vi "Send Command.vi"(8 "error in (no error)":errorcluster, 9 "timeout in ms (0)":i32 format="%d ms", 10 "command":T1={"Command"=enum."Rx", "Parameters"={"arg1"=0, "arg2"=0}}, 11 "Plugin Interface in":refnum<class "Plugin Interface.lvclass">) -> (0 "error out":errorcluster, 3 "Plugin Interface out":refnum<class "Plugin Interface.lvclass">)   [LabVIEW 2021, in "DSF Core.lvlib" / "Plugin Thread.lvclass"]
uses:
  Thread/Plugin/Plugin Thread.lvclass
  Interface/Plugin/Plugin Interface.lvclass
  Interface/Plugin/Command Data.ctl
  Interface/Plugin/Command.ctl
  Interface/Plugin/Command Parameters.ctl
  Interface/Plugin/Send Plugin Command.vi
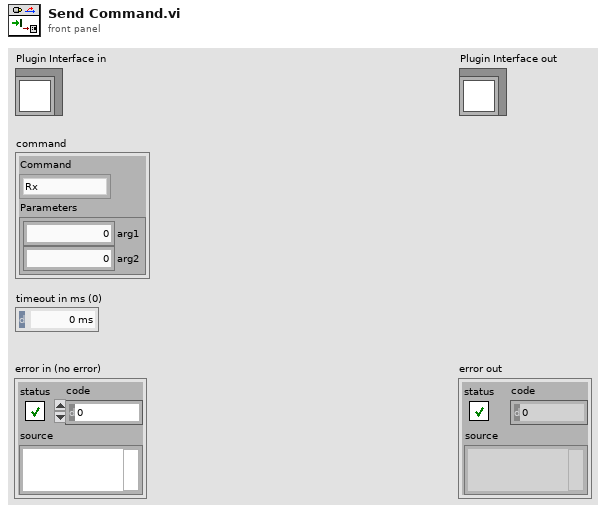
[diagram p1: front panel]
types:
  T1 = typedef "DSF Core.lvlib/Plugin Interface.lvclass/Command Data.ctl" = cluster{"Command":T2, "Parameters":T3}
  T2 = typedef "DSF Core.lvlib/Plugin Interface.lvclass/Command.ctl" = enum8{"Idle", "Start", "Set Inline Buffer", "Rx", "Tx", "Shutdown", "Error"}
  T3 = typedef "DSF Core.lvlib/Plugin Interface.lvclass/Command Parameters.ctl" = cluster{"arg1":u64, "arg2":u64}
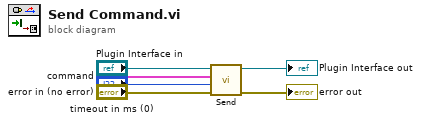
[diagram p0: block diagram]
diagram:
  n1 = call-poly "Send.vi"("error in (no error)"="error in (no error)", "timeout in ms (0)"="timeout in ms (0)", "command"="command", "Plugin Interface in"="Plugin Interface in") -> ("error out"=→"error out":errorcluster, "Plugin Interface out"=→"Plugin Interface out":refnum<class "Plugin Interface.lvclass">)  [unwired: 6 in]
